vi "Set Message.vi"(8 "error in (no error)":errorcluster {"code" format="Error %.0f"}, 10 "Message":string, 11 "g-CLI Interaction in":refnum<class "g-CLI Interaction.lvclass">) -> (0 "error out":errorcluster {"code" format="Error %.0f"}, 3 "g-CLI Interaction out":refnum<class "g-CLI Interaction.lvclass">)   [LabVIEW 2023, in "g-CLI Interaction.lvclass"]
uses:
  g-CLI Interaction.lvclass
  g-CLI Interaction.lvclass/g-CLI Interaction.ctl
  <vilib>/Wiresmith Technology/G CLI/CLI Class/CLI.lvclass
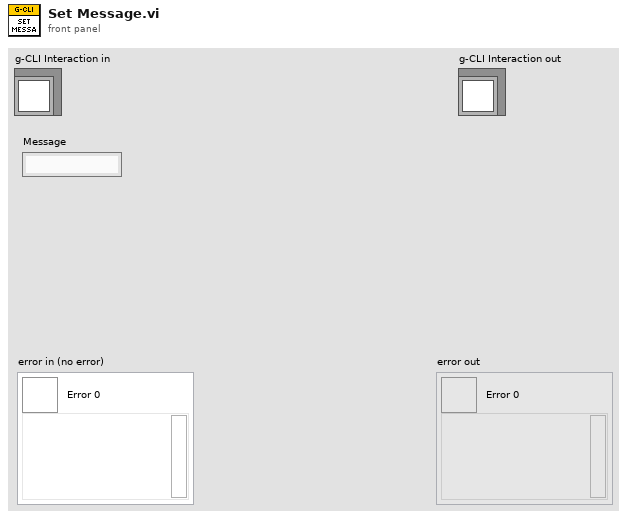
[diagram p1: front panel]
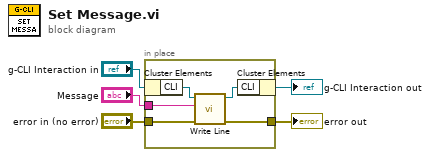
[diagram p0: block diagram]
diagram:
  n1 = in-place {
    in-place-border: "error in (no error)" -> [w8]
    in-place-border: [w7] -> w2
    in-place-border: "Message" -> [w6]
    n2 = in-place-cluster #1("g-CLI Interaction in") -> ("CLI"=w10:refnum<class "CLI.lvclass">)
    n3 = call <vilib>:"Write Line.vi"("error in (no error)"=w8, "Text to Write"=w6, "CLI in"=w10) -> ("error out"=w7:errorcluster, "CLI out"=w9:refnum<class "CLI.lvclass">)  [unwired: 7 in]
    n4 = in-place-cluster #1("CLI"=w9) -> (→"g-CLI Interaction out":refnum<class "g-CLI Interaction.lvclass">)
  }
  "error out" <- w2
